vi "configFileParser.vi"() -> ()   [LabVIEW 2012]
uses:
  <vilib>/Utility/config.llb/Read Key (Double).vi
  <vilib>/Utility/config.llb/NI_LVConfig.lvlib
panel:
  out "armDeadband":dbl
  out "armTwoOtherEnd":dbl
  out "shooterFeederGround":dbl
  out "shooterRPMThreshold":dbl
  out "straightVisionDerivative 2":dbl
  out "straightGyroProportion":dbl
  out "straightGyroIntegral":dbl
  out "straightVisionDerivative":dbl
  out "straightVisionProportion":dbl
  out "straightVisionIntegral":dbl
  out "straightVisionDerivative":dbl
  out "shooterReleaseTiming":dbl
  out "armShooterOnDeadband":dbl
  out "shooterBangBangCeiling":dbl
  out "shooterBangBangFloor":dbl
  out "armLimitLower":dbl
  out "armLimitUpper":dbl
  out "shooterFiringDrop":dbl
  out "shooterQueueFeedingSpeed":dbl
  out "armIntegralCap":dbl
  out "armIntegralDown":dbl
  out "shooterRPMTeleop":dbl
  out "shooterMethod":dbl
  out "armDerivativeUp":dbl
  out "armIntegralUp":dbl
  out "armDerivativeDown":dbl
  out "driveStraightConstant":dbl
  out "armGround":dbl
  out "armTwoPyramidRear":dbl
  out "armFeeder":dbl
  out "armThreePyramidFront":dbl
  out "armThreePyramidRearBlue":dbl
  out "gyroTurnDerivative":dbl
  out "gyroTurnIntegral":dbl
  out "gyroTurnProportion":dbl
  out "cheesySpeedHigh":dbl
  out "cheesySpeedLow":dbl
  out "cheesyQuickHigh":dbl
  out "cheesyQuickLow":dbl
  out "sectionAuto":string[](array[string])
  out "sectionArm":string[](array[string])
  out "sectionDrive":string[](array[string])
  out "sectionShooter":string[](array[string])
  out "shooterDerivative":dbl
  out "shooterIntegral":dbl
  out "shooterProportion":dbl
  out "section names":string[](array[string])
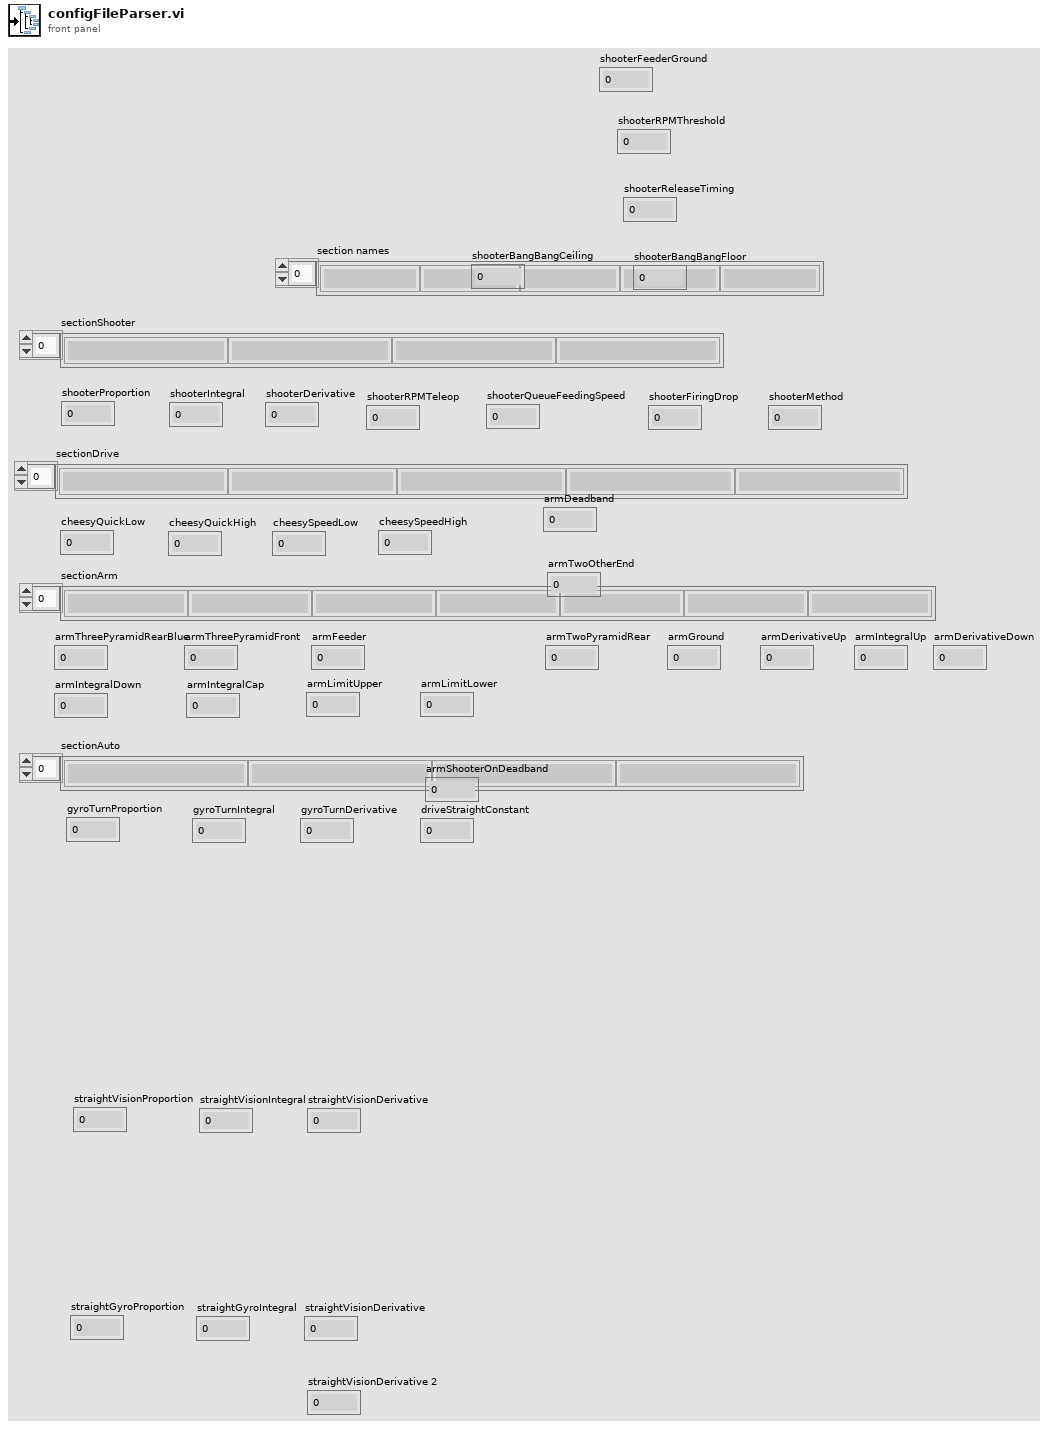
[diagram p1: front panel]
types:
  T1 = typedef "NI_LVConfig.lvlib/Config Data RefNum.ctl" = refnum<k1>
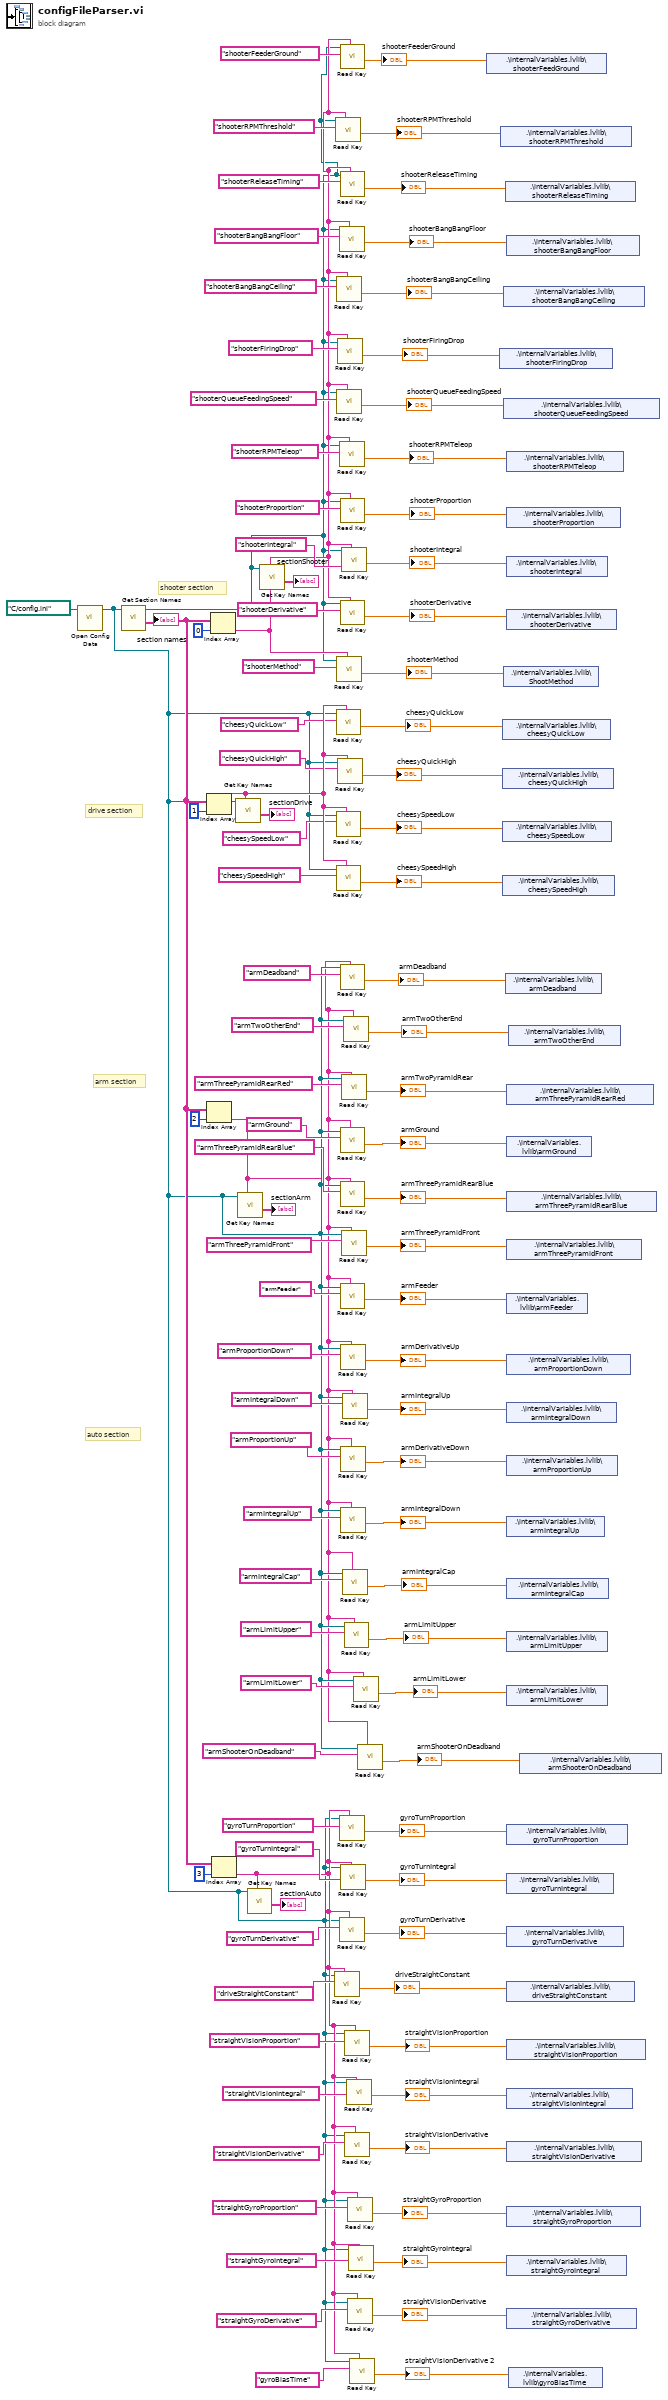
[diagram p0: block diagram]
diagram:
  # "auto section"
  # "arm section"
  # "drive section"
  # "shooter section"
  n1 = call <vilib>:"Open Config Data.vi"("configuration file path"=path "C:/config.ini") -> ("refnum"=w2:T1)  [unwired: 8 in, 2 out]
  n2 = call <vilib>:"Get Section Names.vi"("refnum"=w2) -> ("section names"=w95:string[], "refnum out"=w7:T1)  [unwired: 8 in, 1 out]
  "section names" <- w95
  n3 = Index Array(array=w95, index=1) -> (element=w90:string)
  n4 = Index Array(array=w95, index=2) -> (element=w1:string)
  n5 = Index Array(array=w95, index=0) -> (element=w8:string)
  n6 = Index Array(array=w95, index=3) -> (element=w13:string)
  n7 = call <vilib>:"Get Key Names.vi"("section"=w90, "refnum"=w2) -> ("key names"=→"sectionDrive":string[])  [unwired: 6 in, 3 out]
  n8 = call <vilib>:"Get Key Names.vi"("section"=w1, "refnum"=w2) -> ("key names"=→"sectionArm":string[])  [unwired: 6 in, 3 out]
  n9 = call <vilib>:"Get Key Names.vi"("section"=w13, "refnum"=w2) -> ("key names"=→"sectionAuto":string[])  [unwired: 6 in, 3 out]
  n10 = call <vilib>:"Get Key Names.vi"("section"=w8, "refnum"=w7) -> ("key names"=→"sectionShooter":string[])  [unwired: 6 in, 3 out]
  n11 = call-poly <vilib>:"Read Key.vi"("section"=w13, "key"="driveStraightConstant", "refnum"=w2) -> ("value"=w61:dbl)  [unwired: 5 in, 3 out]
  "driveStraightConstant" <- w61
  n12 = call-poly <vilib>:"Read Key.vi"("section"=w8, "key"="shooterRPMThreshold", "refnum"=w7) -> ("value"=w12:dbl)  [unwired: 5 in, 3 out]
  "shooterRPMThreshold" <- w12
  n13 = call-poly <vilib>:"Read Key.vi"("section"=w90, "key"="cheesyQuickLow", "refnum"=w2) -> ("value"=w66:dbl)  [unwired: 5 in, 3 out]
  "cheesyQuickLow" <- w66
  n14 = call-poly <vilib>:"Read Key.vi"("section"=w90, "key"="cheesySpeedLow", "refnum"=w2) -> ("value"=w64:dbl)  [unwired: 5 in, 3 out]
  "cheesySpeedLow" <- w64
  n15 = call-poly <vilib>:"Read Key.vi"("section"=w90, "key"="cheesySpeedHigh", "refnum"=w2) -> ("value"=w63:dbl)  [unwired: 5 in, 3 out]
  "cheesySpeedHigh" <- w63
  n16 = call-poly <vilib>:"Read Key.vi"("section"=w8, "key"="shooterBangBangCeiling", "refnum"=w7) -> ("value"=w33:dbl)  [unwired: 5 in, 3 out]
  "shooterBangBangCeiling" <- w33
  n17 = call-poly <vilib>:"Read Key.vi"("section"=w8, "key"="shooterQueueFeedingSpeed", "refnum"=w7) -> ("value"=w42:dbl)  [unwired: 5 in, 3 out]
  "shooterQueueFeedingSpeed" <- w42
  n18 = call-poly <vilib>:"Read Key.vi"("section"=w8, "key"="shooterMethod", "refnum"=w7) -> ("value"=w51:dbl)  [unwired: 5 in, 3 out]
  "shooterMethod" <- w51
  n19 = call-poly <vilib>:"Read Key.vi"("section"=w8, "key"="shooterFiringDrop", "refnum"=w7) -> ("value"=w41:dbl)  [unwired: 5 in, 3 out]
  "shooterFiringDrop" <- w41
  n20 = call-poly <vilib>:"Read Key.vi"("section"=w90, "key"="cheesyQuickHigh", "refnum"=w2) -> ("value"=w65:dbl)  [unwired: 5 in, 3 out]
  "cheesyQuickHigh" <- w65
  n21 = call-poly <vilib>:"Read Key.vi"("section"=w8, "key"="shooterBangBangFloor", "refnum"=w7) -> ("value"=w34:dbl)  [unwired: 5 in, 3 out]
  "shooterBangBangFloor" <- w34
  n22 = call-poly <vilib>:"Read Key.vi"("section"=w8, "key"="shooterRPMTeleop", "refnum"=w7) -> ("value"=w49:dbl)  [unwired: 5 in, 3 out]
  "shooterRPMTeleop" <- w49
  n23 = call-poly <vilib>:"Read Key.vi"("section"=w13, "key"="gyroTurnProportion", "refnum"=w2) -> ("value"=w58:dbl)  [unwired: 5 in, 3 out]
  "gyroTurnProportion" <- w58
  n24 = call-poly <vilib>:"Read Key.vi"("section"=w13, "key"="gyroTurnDerivative", "refnum"=w2) -> ("value"=w60:dbl)  [unwired: 5 in, 3 out]
  "gyroTurnDerivative" <- w60
  n25 = call-poly <vilib>:"Read Key.vi"("section"=w8, "key"="shooterFeederGround", "refnum"=w7) -> ("value"=w9:dbl)  [unwired: 5 in, 3 out]
  "shooterFeederGround" <- w9
  n26 = call-poly <vilib>:"Read Key.vi"("section"=w8, "key"="shooterReleaseTiming", "refnum"=w7) -> ("value"=w28:dbl)  [unwired: 5 in, 3 out]
  "shooterReleaseTiming" <- w28
  n27 = call-poly <vilib>:"Read Key.vi"("section"=w8, "key"="shooterProportion", "refnum"=w7) -> ("value"=w69:dbl)  [unwired: 5 in, 3 out]
  "shooterProportion" <- w69
  n28 = call-poly <vilib>:"Read Key.vi"("section"=w8, "key"="shooterDerivative", "refnum"=w7) -> ("value"=w67:dbl)  [unwired: 5 in, 3 out]
  "shooterDerivative" <- w67
  n29 = call-poly <vilib>:"Read Key.vi"("section"=w1, "key"="armDeadband", "refnum"=w2) -> ("value"=w3:dbl)  [unwired: 5 in, 3 out]
  "armDeadband" <- w3
  n30 = call-poly <vilib>:"Read Key.vi"("section"=w1, "key"="armGround", "refnum"=w2) -> ("value"=w72:dbl)  [unwired: 5 in, 3 out]
  "armGround" <- w72
  n31 = call-poly <vilib>:"Read Key.vi"("section"=w1, "key"="armThreePyramidRearBlue", "refnum"=w2) -> ("value"=w73:dbl)  [unwired: 5 in, 3 out]
  "armThreePyramidRearBlue" <- w73
  n32 = call-poly <vilib>:"Read Key.vi"("section"=w1, "key"="armFeeder", "refnum"=w2) -> ("value"=w74:dbl)  [unwired: 5 in, 3 out]
  "armFeeder" <- w74
  n33 = call-poly <vilib>:"Read Key.vi"("section"=w1, "key"="armProportionDown", "refnum"=w2) -> ("value"=w57:dbl)  [unwired: 5 in, 3 out]
  "armDerivativeUp" <- w57
  n34 = call-poly <vilib>:"Read Key.vi"("section"=w1, "key"="armProportionUp", "refnum"=w2) -> ("value"=w55:dbl)  [unwired: 5 in, 3 out]
  "armDerivativeDown" <- w55
  n35 = call-poly <vilib>:"Read Key.vi"("section"=w1, "key"="armIntegralUp", "refnum"=w2) -> ("value"=w46:dbl)  [unwired: 5 in, 3 out]
  "armIntegralDown" <- w46
  n36 = call-poly <vilib>:"Read Key.vi"("section"=w13, "key"="gyroTurnIntegral", "refnum"=w2) -> ("value"=w59:dbl)  [unwired: 5 in, 3 out]
  "gyroTurnIntegral" <- w59
  n37 = call-poly <vilib>:"Read Key.vi"("section"=w8, "key"="shooterIntegral", "refnum"=w7) -> ("value"=w68:dbl)  [unwired: 5 in, 3 out]
  "shooterIntegral" <- w68
  n38 = call-poly <vilib>:"Read Key.vi"("section"=w1, "key"="armThreePyramidRearRed", "refnum"=w2) -> ("value"=w71:dbl)  [unwired: 5 in, 3 out]
  "armTwoPyramidRear" <- w71
  n39 = call-poly <vilib>:"Read Key.vi"("section"=w1, "key"="armThreePyramidFront", "refnum"=w2) -> ("value"=w70:dbl)  [unwired: 5 in, 3 out]
  "armThreePyramidFront" <- w70
  n40 = call-poly <vilib>:"Read Key.vi"("section"=w1, "key"="armIntegralDown", "refnum"=w2) -> ("value"=w56:dbl)  [unwired: 5 in, 3 out]
  "armIntegralUp" <- w56
  n41 = call-poly <vilib>:"Read Key.vi"("section"=w1, "key"="armIntegralCap", "refnum"=w2) -> ("value"=w45:dbl)  [unwired: 5 in, 3 out]
  "armIntegralCap" <- w45
  n42 = call-poly <vilib>:"Read Key.vi"("section"=w1, "key"="armTwoOtherEnd", "refnum"=w2) -> ("value"=w6:dbl)  [unwired: 5 in, 3 out]
  "armTwoOtherEnd" <- w6
  n43 = call-poly <vilib>:"Read Key.vi"("section"=w1, "key"="armLimitUpper", "refnum"=w2) -> ("value"=w36:dbl)  [unwired: 5 in, 3 out]
  "armLimitUpper" <- w36
  n44 = call-poly <vilib>:"Read Key.vi"("section"=w13, "key"="straightVisionProportion", "refnum"=w2) -> ("value"=w24:dbl)  [unwired: 5 in, 3 out]
  "straightVisionProportion" <- w24
  n45 = call-poly <vilib>:"Read Key.vi"("section"=w13, "key"="straightVisionDerivative", "refnum"=w2) -> ("value"=w17:dbl)  [unwired: 5 in, 3 out]
  "straightVisionDerivative" <- w17
  n46 = call-poly <vilib>:"Read Key.vi"("section"=w13, "key"="straightVisionIntegral", "refnum"=w2) -> ("value"=w16:dbl)  [unwired: 5 in, 3 out]
  "straightVisionIntegral" <- w16
  n47 = call-poly <vilib>:"Read Key.vi"("section"=w13, "key"="straightGyroProportion", "refnum"=w2) -> ("value"=w18:dbl)  [unwired: 5 in, 3 out]
  "straightGyroProportion" <- w18
  n48 = call-poly <vilib>:"Read Key.vi"("section"=w13, "key"="straightGyroDerivative", "refnum"=w2) -> ("value"=w20:dbl)  [unwired: 5 in, 3 out]
  "straightVisionDerivative" <- w20
  n49 = call-poly <vilib>:"Read Key.vi"("section"=w13, "key"="straightGyroIntegral", "refnum"=w2) -> ("value"=w19:dbl)  [unwired: 5 in, 3 out]
  "straightGyroIntegral" <- w19
  n50 = call-poly <vilib>:"Read Key.vi"("section"=w13, "key"="gyroBiasTime", "refnum"=w2) -> ("value"=w15:dbl)  [unwired: 5 in, 3 out]
  "straightVisionDerivative 2" <- w15
  n51 = call-poly <vilib>:"Read Key.vi"("section"=w1, "key"="armLimitLower", "refnum"=w2) -> ("value"=w37:dbl)  [unwired: 5 in, 3 out]
  "armLimitLower" <- w37
  n52 = call-poly <vilib>:"Read Key.vi"("section"=w1, "key"="armShooterOnDeadband", "refnum"=w2) -> ("value"=w30:dbl)  [unwired: 5 in, 3 out]
  "armShooterOnDeadband" <- w30
  n53 = shared-variable ".\\internalVariables.lvlib\\shooterFeedGround"(w9) -> ()  [unwired: 1 in, 1 out]
  n54 = shared-variable ".\\internalVariables.lvlib\\shooterFiringDrop"(w41) -> ()  [unwired: 1 in, 1 out]
  n55 = shared-variable ".\\internalVariables.lvlib\\shooterRPMThreshold"(w12) -> ()  [unwired: 1 in, 1 out]
  n56 = shared-variable ".\\internalVariables.lvlib\\cheesyQuickLow"(w66) -> ()  [unwired: 1 in, 1 out]
  n57 = shared-variable ".\\internalVariables.lvlib\\cheesyQuickHigh"(w65) -> ()  [unwired: 1 in, 1 out]
  n58 = shared-variable ".\\internalVariables.lvlib\\cheesySpeedLow"(w64) -> ()  [unwired: 1 in, 1 out]
  n59 = shared-variable ".\\internalVariables.lvlib\\cheesySpeedHigh"(w63) -> ()  [unwired: 1 in, 1 out]
  n60 = shared-variable ".\\internalVariables.lvlib\\shooterBangBangCeiling"(w33) -> ()  [unwired: 1 in, 1 out]
  n61 = shared-variable ".\\internalVariables.lvlib\\shooterQueueFeedingSpeed"(w42) -> ()  [unwired: 1 in, 1 out]
  n62 = shared-variable ".\\internalVariables.lvlib\\ShootMethod"(w51) -> ()  [unwired: 1 in, 1 out]
  n63 = shared-variable ".\\internalVariables.lvlib\\shooterReleaseTiming"(w28) -> ()  [unwired: 1 in, 1 out]
  n64 = shared-variable ".\\internalVariables.lvlib\\armDeadband"(w3) -> ()  [unwired: 1 in, 1 out]
  n65 = shared-variable ".\\internalVariables.lvlib\\shooterBangBangFloor"(w34) -> ()  [unwired: 1 in, 1 out]
  n66 = shared-variable ".\\internalVariables.lvlib\\shooterRPMTeleop"(w49) -> ()  [unwired: 1 in, 1 out]
  n67 = shared-variable ".\\internalVariables.lvlib\\gyroTurnProportion"(w58) -> ()  [unwired: 1 in, 1 out]
  n68 = shared-variable ".\\internalVariables.lvlib\\gyroTurnIntegral"(w59) -> ()  [unwired: 1 in, 1 out]
  n69 = shared-variable ".\\internalVariables.lvlib\\gyroTurnDerivative"(w60) -> ()  [unwired: 1 in, 1 out]
  n70 = shared-variable ".\\internalVariables.lvlib\\driveStraightConstant"(w61) -> ()  [unwired: 1 in, 1 out]
  n71 = shared-variable ".\\internalVariables.lvlib\\straightVisionProportion"(w24) -> ()  [unwired: 1 in, 1 out]
  n72 = shared-variable ".\\internalVariables.lvlib\\straightVisionIntegral"(w16) -> ()  [unwired: 1 in, 1 out]
  n73 = shared-variable ".\\internalVariables.lvlib\\straightVisionDerivative"(w17) -> ()  [unwired: 1 in, 1 out]
  n74 = shared-variable ".\\internalVariables.lvlib\\straightGyroProportion"(w18) -> ()  [unwired: 1 in, 1 out]
  n75 = shared-variable ".\\internalVariables.lvlib\\straightGyroIntegral"(w19) -> ()  [unwired: 1 in, 1 out]
  n76 = shared-variable ".\\internalVariables.lvlib\\straightGyroDerivative"(w20) -> ()  [unwired: 1 in, 1 out]
  n77 = shared-variable ".\\internalVariables.lvlib\\shooterProportion"(w69) -> ()  [unwired: 1 in, 1 out]
  n78 = shared-variable ".\\internalVariables.lvlib\\shooterIntegral"(w68) -> ()  [unwired: 1 in, 1 out]
  n79 = shared-variable ".\\internalVariables.lvlib\\shooterDerivative"(w67) -> ()  [unwired: 1 in, 1 out]
  n80 = shared-variable ".\\internalVariables.lvlib\\armThreePyramidRearRed"(w71) -> ()  [unwired: 1 in, 1 out]
  n81 = shared-variable ".\\internalVariables.lvlib\\armGround"(w72) -> ()  [unwired: 1 in, 1 out]
  n82 = shared-variable ".\\internalVariables.lvlib\\armThreePyramidRearBlue"(w73) -> ()  [unwired: 1 in, 1 out]
  n83 = shared-variable ".\\internalVariables.lvlib\\armThreePyramidFront"(w70) -> ()  [unwired: 1 in, 1 out]
  n84 = shared-variable ".\\internalVariables.lvlib\\armFeeder"(w74) -> ()  [unwired: 1 in, 1 out]
  n85 = shared-variable ".\\internalVariables.lvlib\\armProportionDown"(w57) -> ()  [unwired: 1 in, 1 out]
  n86 = shared-variable ".\\internalVariables.lvlib\\armIntegralDown"(w56) -> ()  [unwired: 1 in, 1 out]
  n87 = shared-variable ".\\internalVariables.lvlib\\armProportionUp"(w55) -> ()  [unwired: 1 in, 1 out]
  n88 = shared-variable ".\\internalVariables.lvlib\\armIntegralUp"(w46) -> ()  [unwired: 1 in, 1 out]
  n89 = shared-variable ".\\internalVariables.lvlib\\armIntegralCap"(w45) -> ()  [unwired: 1 in, 1 out]
  n90 = shared-variable ".\\internalVariables.lvlib\\armLimitUpper"(w36) -> ()  [unwired: 1 in, 1 out]
  n91 = shared-variable ".\\internalVariables.lvlib\\armLimitLower"(w37) -> ()  [unwired: 1 in, 1 out]
  n92 = shared-variable ".\\internalVariables.lvlib\\armTwoOtherEnd"(w6) -> ()  [unwired: 1 in, 1 out]
  n93 = shared-variable ".\\internalVariables.lvlib\\gyroBiasTime"(w15) -> ()  [unwired: 1 in, 1 out]
  n94 = shared-variable ".\\internalVariables.lvlib\\armShooterOnDeadband"(w30) -> ()  [unwired: 1 in, 1 out]
